vi "ConvertToFlanks10.vi"(10 "10bit input":bool[](array[boolean])=[FALSE, FALSE, FALSE, FALSE, FALSE, FALSE, FALSE, FALSE, FALSE, FALSE], 11 "Last sample in":bool=TRUE) -> (2 "Flank output":bool[](array[boolean]), 3 "Last sample out":bool=TRUE)   [LabVIEW 2012]
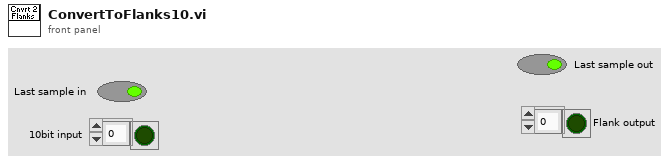
[diagram p1: front panel]
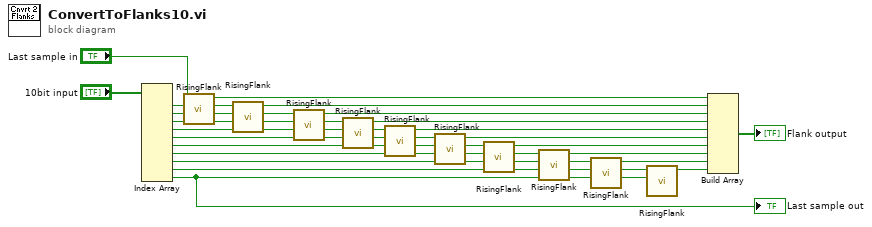
[diagram p0: block diagram]
diagram:
  n1 = Index Array(array="10bit input") -> (element #1=w21:bool, element #2=w20:bool, element #3=w19:bool, element #4=w18:bool, element #5=w17:bool, element #6=w16:bool, element #7=w15:bool, element #8=w14:bool, element #9=w13:bool, element #10=w12:bool)  [unwired: 10 in]
  "Last sample out" <- w12
  n2 = call "RisingFlank.vi"("2nd sample"=w21, "1st sample"="Last sample in") -> ("Rising flank?"=w11:bool)  [unwired: 7 in]
  n3 = call "RisingFlank.vi"("2nd sample"=w20, "1st sample"=w21) -> ("Rising flank?"=w10:bool)  [unwired: 7 in]
  n4 = call "RisingFlank.vi"("2nd sample"=w19, "1st sample"=w20) -> ("Rising flank?"=w9:bool)  [unwired: 7 in]
  n5 = call "RisingFlank.vi"("2nd sample"=w18, "1st sample"=w19) -> ("Rising flank?"=w8:bool)  [unwired: 7 in]
  n6 = call "RisingFlank.vi"("2nd sample"=w17, "1st sample"=w18) -> ("Rising flank?"=w7:bool)  [unwired: 7 in]
  n7 = call "RisingFlank.vi"("2nd sample"=w16, "1st sample"=w17) -> ("Rising flank?"=w6:bool)  [unwired: 7 in]
  n8 = call "RisingFlank.vi"("2nd sample"=w15, "1st sample"=w16) -> ("Rising flank?"=w5:bool)  [unwired: 7 in]
  n9 = call "RisingFlank.vi"("2nd sample"=w14, "1st sample"=w15) -> ("Rising flank?"=w4:bool)  [unwired: 7 in]
  n10 = call "RisingFlank.vi"("2nd sample"=w13, "1st sample"=w14) -> ("Rising flank?"=w3:bool)  [unwired: 7 in]
  n11 = call "RisingFlank.vi"("2nd sample"=w12, "1st sample"=w13) -> ("Rising flank?"=w2:bool)  [unwired: 7 in]
  n12 = Build Array(w11, w10, w9, w8, w7, w6, w5, w4, w3, w2) -> (→"Flank output":bool[])
